vi "3D-Cal_Flatness.vi"(9 "Ratid":dbl, 10 "坐标输入":string[](array[string]), 11 "pic z value":dbl[][](array[numeric])) -> (0 "Base Poit":cluster{"X":dbl, "Y":dbl, "Z":dbl}[](array[cluster]), 1 "添加的数组":cluster{"X":dbl, "Y":dbl, "Z":dbl}[](array[cluster]), 2 "Z":string[](array[string]), 3 "Max Center XY":cluster{"X":dbl, "Y":dbl})   [LabVIEW 2015]
panel:
  in  "索引 2":i32
  out "索引":i32
  out "波形图":dbl[](graph)
  in  "索引 (行)":i32
  out "Y":i32[](array[numeric])
  out "X":i32[](array[numeric])
  # "0 Left\n1 Top\n2 Right\n3 Bottom\n4 p1 Center\n5 p2 Center\n6 P3 Center\n7 p4 Center"
  # "行值"
  # "列值"
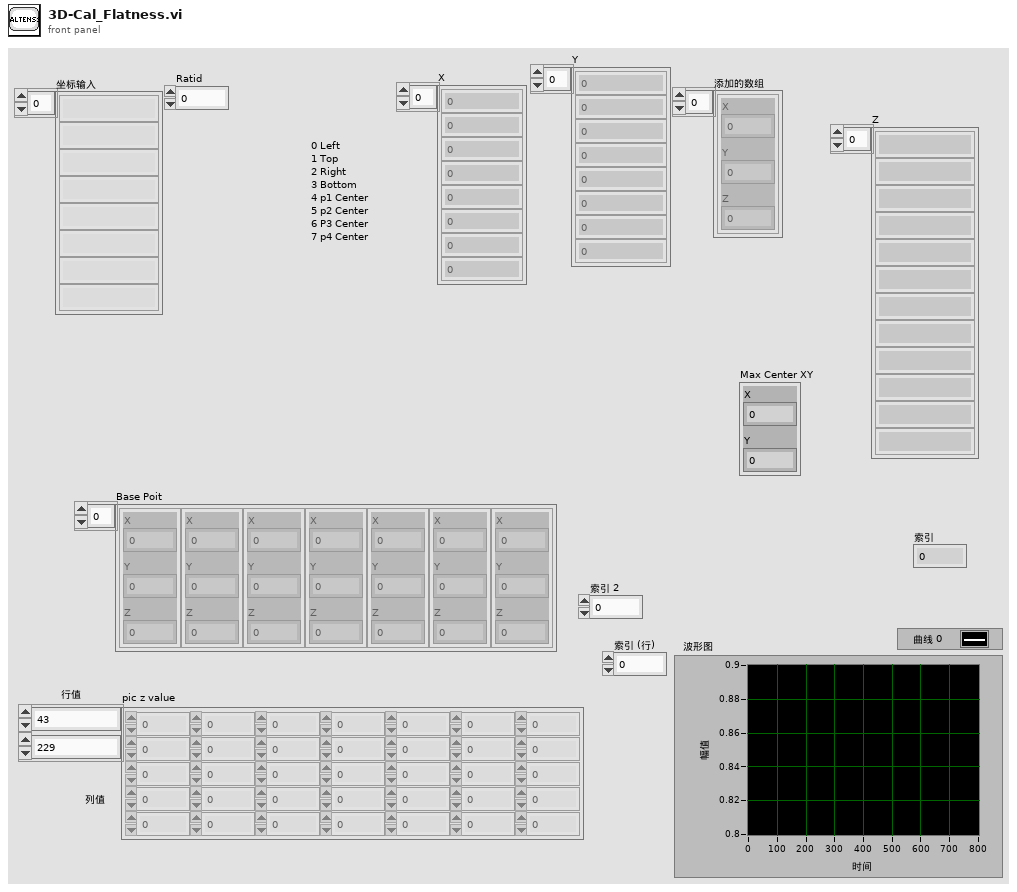
[diagram p1: front panel]
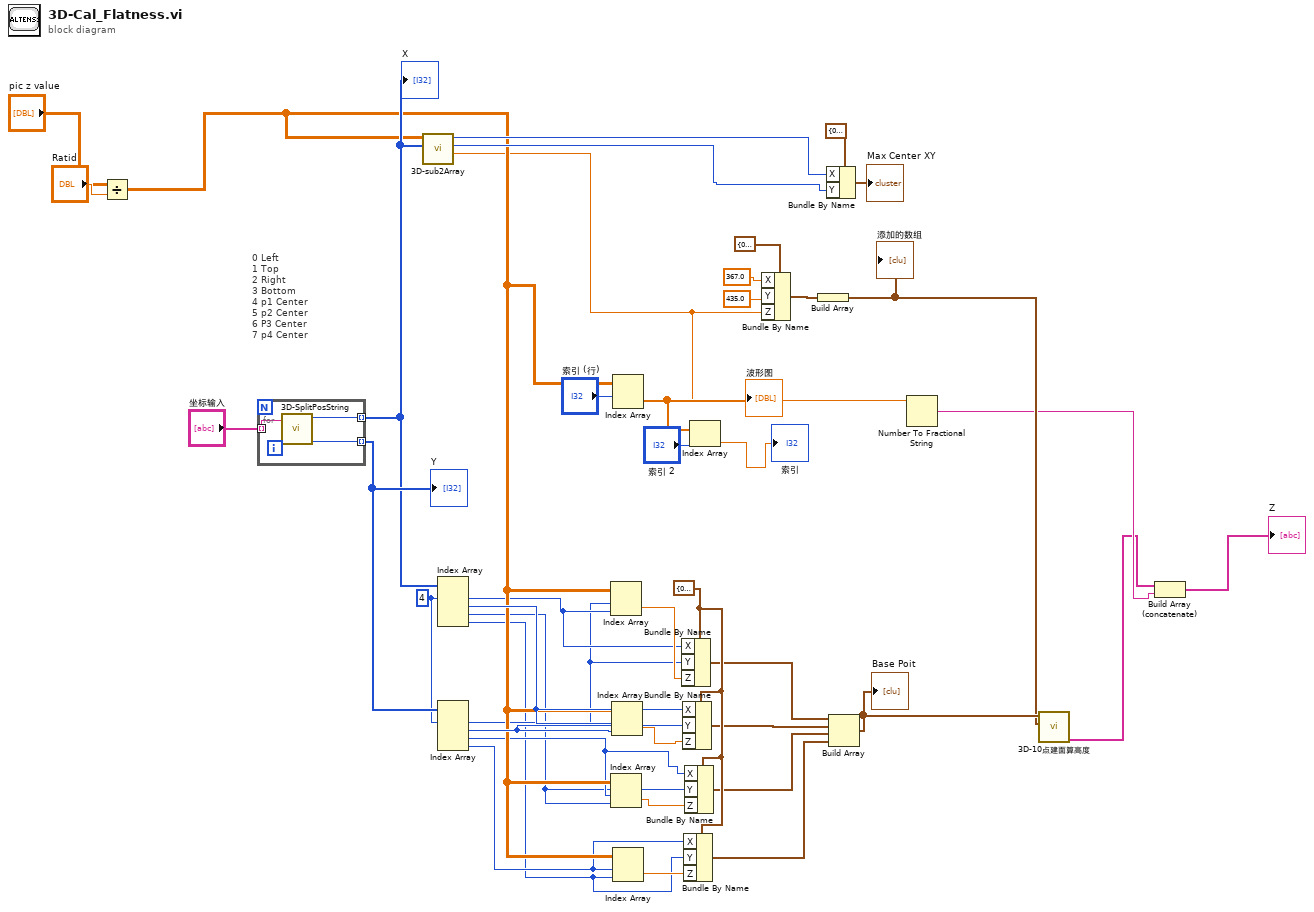
[diagram p0: block diagram]
diagram:
  w33 = cluster{"X":dbl, "Y":dbl, "Z":dbl} {"X"=0.0, "Y"=0.0, "Z"=0.0} ("输入簇")
  w40 = 4 ("索引")
  # "0 Left\n1 Top\n2 Right\n3 Bottom\n4 p1 Center\n5 p2 Center\n6 P3 Center\n7 p4 Center"
  n1 = Divide(x="pic z value", y="Ratid") -> (x/y=w13:dbl[][])
  n2 = for {
    tunnel: "坐标输入" -> [w45] mode=indexing
    tunnel: [w44] -> w18 mode=indexing
    tunnel: [w43] -> w41 mode=indexing
    n3 = call "3D-SplitPosString.vi"("input pos array"=w45) -> ("Y pos"=w43:i32, "X pos"=w44:i32)  [unwired: 7 in, 2 out]
  }
  "X" <- w18
  "Y" <- w41
  n4 = call "3D-sub2Array.vi"("X"=w18, "pic z value"=w13) -> ("最大值"=w12:dbl, "行值"=w16:i32, "列值"=w17:i32)  [unwired: 7 in]
  n5 = Index Array(array=w18, index #1=w40) -> (element #1=w8:i32, element #2=w38:i32, element #3=w5:i32, element #4=w3:i32)  [unwired: 3 in]
  n6 = Index Array(array=w41, index #1=w40) -> (element #1=w7:i32, element #2=w37:i32, element #3=w6:i32, element #4=w4:i32)  [unwired: 3 in]
  n7 = Index Array(array=w13, index (row)=w7, index (col)=w8) -> (element=w39:dbl)
  n8 = Index Array(array=w13, index (row)=w6, index (col)=w5) -> (element=w35:dbl)
  n9 = Index Array(array=w13, index (row)=w38, index (col)=w37) -> (element=w36:dbl)
  n10 = Index Array(array=w13, index (row)="索引 (行)") -> (element=w21:dbl[])  [unwired: 1 in]
  "波形图" <- w21
  n11 = Index Array(array=w13, index (row)=w4, index (col)=w3) -> (element=w34:dbl)
  n12 = Bundle By Name(cluster=w33, "X"=w8, "Y"=w7, "Z"=w39) -> (w32:cluster{"X":dbl, "Y":dbl, "Z":dbl})
  n13 = Bundle By Name(cluster=w33, "X"=w38, "Y"=w37, "Z"=w36) -> (w31:cluster{"X":dbl, "Y":dbl, "Z":dbl})
  n14 = Bundle By Name(cluster=w33, "X"=w4, "Y"=w3, "Z"=w34) -> (w29:cluster{"X":dbl, "Y":dbl, "Z":dbl})
  n15 = Bundle By Name(cluster=w33, "X"=w6, "Y"=w5, "Z"=w35) -> (w30:cluster{"X":dbl, "Y":dbl, "Z":dbl})
  n16 = Index Array(array=w21, index="索引 2") -> (element=→"索引":dbl)
  n17 = Bundle By Name(cluster=cluster{"X":dbl, "Y":dbl, "Z":dbl} {"X"=0.0, "Y"=0.0, "Z"=0.0} ("输入簇"), "X"=367.0, "Y"=435.0, "Z"=w12) -> (w26:cluster{"X":dbl, "Y":dbl, "Z":dbl})
  n18 = Build Array(w26) -> (w25:cluster{"X":dbl, "Y":dbl, "Z":dbl}[])
  "添加的数组" <- w25
  n19 = Bundle By Name(cluster=cluster{"X":dbl, "Y":dbl} {"X"=0.0, "Y"=0.0} ("输入簇"), "X"=w17, "Y"=w16) -> (→"Max Center XY":cluster{"X":dbl, "Y":dbl})
  n20 = Build Array(w32, w31, w30, w29) -> (w28:cluster{"X":dbl, "Y":dbl, "Z":dbl}[])
  "Base Poit" <- w28
  n21 = Number To Fractional String(number=w12) -> (F-format string=w11:string)  [unwired: 3 in]
  n22 = call "3D-10点建面算高度.vi"("Max 位置数组"=w25, "基准点数组"=w28) -> ("Z"=w10:string[])  [unwired: 8 in, 1 out]
  n23 = Build Array (concatenate)(w10, w11) -> (→"Z":string[])
